vi "Maquina de Estados Basica.vi"() -> ()   [LabVIEW 2016]
panel:
  out "Estado 5":bool
  out "Estado 4":bool
  out "Estado 3":bool
  out "Estado 2":bool
  out "Estado 1":bool
  in  "Anterior":bool
  in  "Siguiente":bool
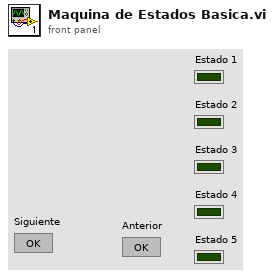
[diagram p1: front panel]
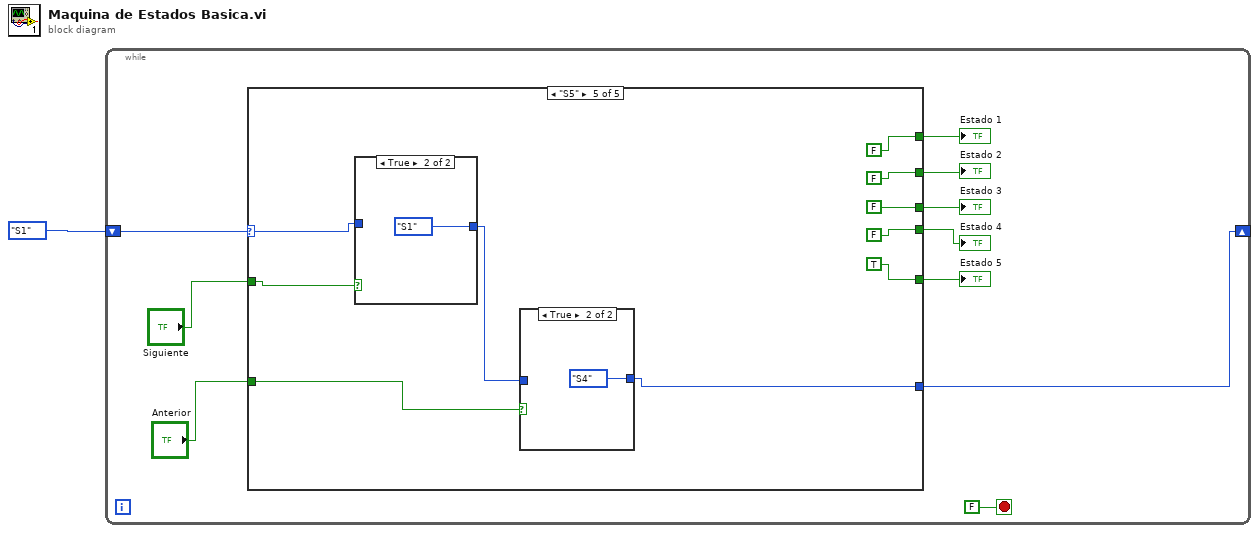
[diagram p0: block diagram]
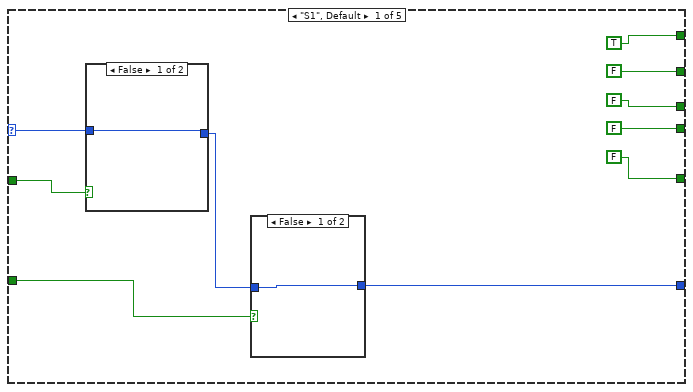
[diagram p2: hidden frame]
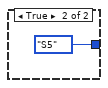
[diagram p3: hidden frame]
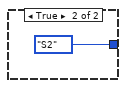
[diagram p4: hidden frame]
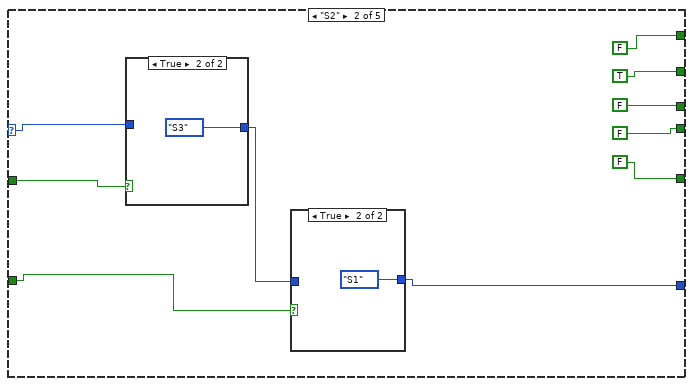
[diagram p5: hidden frame]
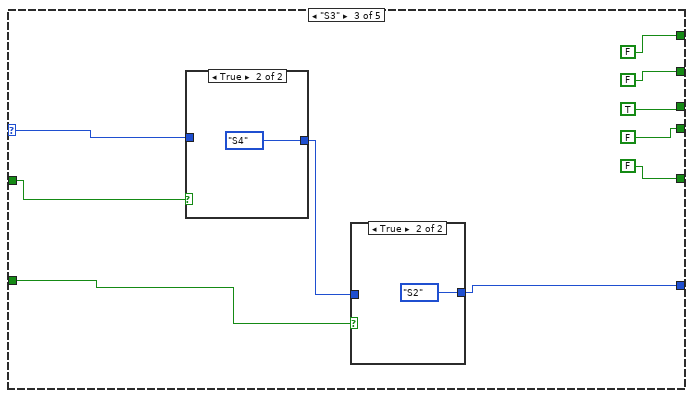
[diagram p8: hidden frame]
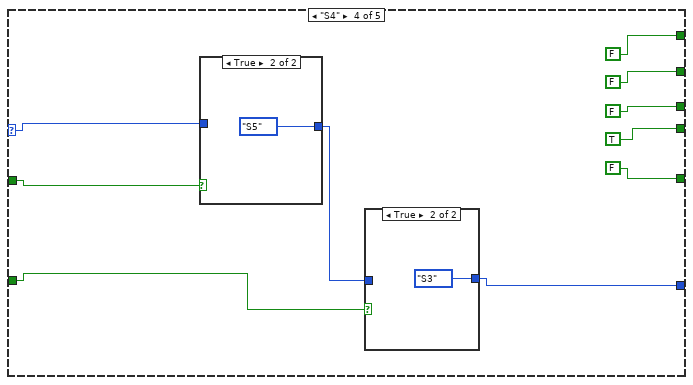
[diagram p11: hidden frame]
diagram:
  n1 = while {
    shift-right: [w2] -> _
    shift-left: enum16{"S1", "S2", "S3", "S4", "S5"}."S1" -> [w10]
    stop <- FALSE stop-if-true
    n2 = case shown="\"S5\"" w10 {
      selector: w10 -> [w15 w27 w43 w57 w71]
      tunnel: [TRUE FALSE FALSE FALSE FALSE] -> w9
      tunnel: [FALSE TRUE FALSE FALSE FALSE] -> w8
      tunnel: [FALSE FALSE TRUE FALSE FALSE] -> w7
      tunnel: [FALSE FALSE FALSE TRUE FALSE] -> w6
      tunnel: [FALSE FALSE FALSE FALSE TRUE] -> w5
      tunnel: "Siguiente" -> [w16 w29 w41 w54 w69]
      tunnel: "Anterior" -> [w14 w28 w42 w55 w70]
      tunnel: [w12 w26 w40 w56 w68] -> w2
      frame "S1", Default {
        n3 = case shown="False" w16 {
          tunnel: w15 -> [w24 _]
          tunnel: [w24 enum16{"S1", "S2", "S3", "S4", "S5"}."S2"] -> w13
          frame False {
          }
          frame True {
          }
        }
        n4 = case shown="False" w14 {
          tunnel: [w22 enum16{"S1", "S2", "S3", "S4", "S5"}."S5"] -> w12
          tunnel: w13 -> [w22 _]
          frame False {
          }
          frame True {
          }
        }
      }
      frame "S2" {
        n5 = case shown="True" w29 {
          tunnel: w27 -> [w38 _]
          tunnel: [w38 enum16{"S1", "S2", "S3", "S4", "S5"}."S3"] -> w30
          frame False {
          }
          frame True {
          }
        }
        n6 = case shown="True" w28 {
          tunnel: [w36 enum16{"S1", "S2", "S3", "S4", "S5"}."S1"] -> w26
          tunnel: w30 -> [w36 _]
          frame False {
          }
          frame True {
          }
        }
      }
      frame "S3" {
        n7 = case shown="True" w41 {
          tunnel: w43 -> [w52 _]
          tunnel: [w52 enum16{"S1", "S2", "S3", "S4", "S5"}."S4"] -> w44
          frame False {
          }
          frame True {
          }
        }
        n8 = case shown="True" w42 {
          tunnel: [w50 enum16{"S1", "S2", "S3", "S4", "S5"}."S2"] -> w40
          tunnel: w44 -> [w50 _]
          frame False {
          }
          frame True {
          }
        }
      }
      frame "S4" {
        n9 = case shown="True" w54 {
          tunnel: w57 -> [w66 _]
          tunnel: [w66 enum16{"S1", "S2", "S3", "S4", "S5"}."S5"] -> w58
          frame False {
          }
          frame True {
          }
        }
        n10 = case shown="True" w55 {
          tunnel: [w64 enum16{"S1", "S2", "S3", "S4", "S5"}."S3"] -> w56
          tunnel: w58 -> [w64 _]
          frame False {
          }
          frame True {
          }
        }
      }
      frame "S5" {
        n11 = case shown="True" w69 {
          tunnel: w71 -> [w80 _]
          tunnel: [w80 enum16{"S1", "S2", "S3", "S4", "S5"}."S1"] -> w72
          frame False {
          }
          frame True {
          }
        }
        n12 = case shown="True" w70 {
          tunnel: [w78 enum16{"S1", "S2", "S3", "S4", "S5"}."S4"] -> w68
          tunnel: w72 -> [w78 _]
          frame False {
          }
          frame True {
          }
        }
      }
    }
    "Estado 2" <- w8
    "Estado 1" <- w9
    "Estado 3" <- w7
    "Estado 4" <- w6
    "Estado 5" <- w5
  }
